vi "LVClass_SlopesPostProcessList GetParameter_DoublePassage.vi"(0 "SlopesPostProcessorList in":refnum<class "SlopesPostProcessorList.lvclass">, 5 "Position":u32, 11 "error in (no error)":errorcluster) -> (4 "SlopesPostProcessorList out":refnum<class "SlopesPostProcessorList.lvclass">, 8 "doublePath":T1, 15 "error out":errorcluster)   [LabVIEW 2020, in "SlopesPostProcessorList.lvclass"]
doc: "Get parameters of the DoublePath processor.\n\n--------------------------------------------------------------------------------\n\n<B>SlopesPostProcessorListIn </B> : SlopesPostProcessorList object.\n<B>SlopesPostProcessorListOut </B> : SlopesPostProcessorList object.\n<B>position </B> : Position of the processor in the SlopesPostProcessorList.\n<B>DoublePathActivateOnTilt </B> : State of Double path activation on tilt.\n<B>DoublePathActivateOnCurvature</B> : State of Double path activation on curvature.\n<B>ErrorIn </B> : Error\n<B>ErrorOut </B> : Error\n\n--------------------------------------------------------------------------------"
uses:
  SlopesPostProcessorList.lvclass
  Controls/SlopesPostProcessorList - Double passage.ctl
  SlopesPostProcessorList.lvclass/SlopesPostProcessorList.ctl
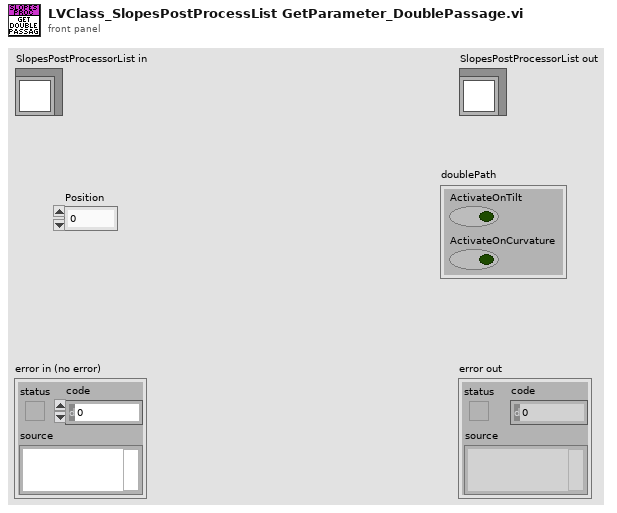
[diagram p1: front panel]
types:
  T1 = typedef "SlopesPostProcessorList - Double passage.ctl" = cluster{"ActivateOnTilt":bool, "ActivateOnCurvature":bool}
  T2 = typedef "ClassID.ctl" = i64
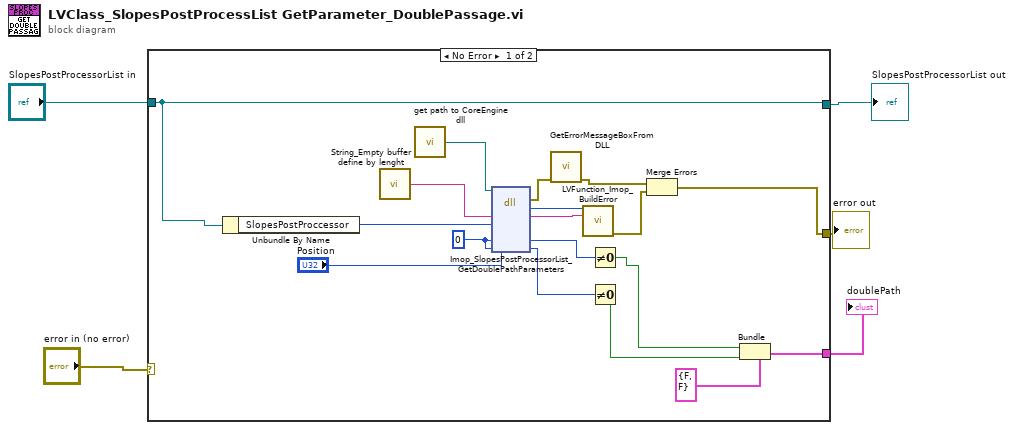
[diagram p0: block diagram]
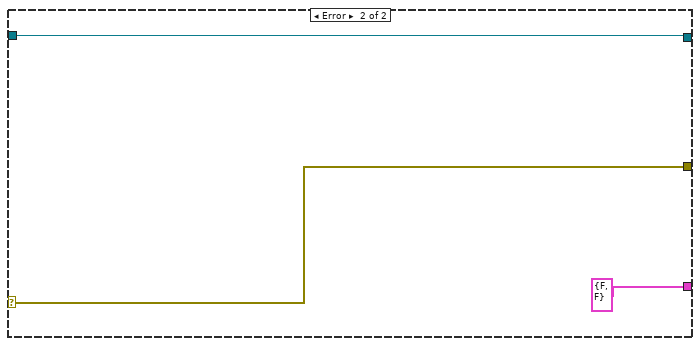
[diagram p2: hidden frame]
diagram:
  n1 = case shown="No Error" "error in (no error)" {
    selector: "error in (no error)" -> [_ w25]
    tunnel: "SlopesPostProcessorList in" -> [w18 w26]
    tunnel: [w18 w26] -> w3
    tunnel: [w10 w25] -> w2
    tunnel: [w7 T1 {"ActivateOnTilt"=FALSE, "ActivateOnCurvature"=FALSE} ("doublePassage")] -> w1
    frame No Error {
      w16 = u8 0 ("doublePassageActivateOnTilt")
      n2 = Unbundle By Name(w18) -> ("SlopesPostProccessor"=w17:T2)
      n3 = call "String_Empty buffer define by lenght.vi"() -> ("Empty buffer"=w23:string)  [unwired: 1 in]
      n4 = call "get path to CoreEngine dll.vi"() -> ("path to wavekit library"=w20:path)  [unwired: 14 in, 1 out]
      n5 = dll-call lib="D:/soft/HASO_v3/SVN_trunk/ImOpCoreEngine4_LV2011/DLLs/c_interface_vc100.dll" fn="Imop_SlopesPostProcessorList_GetDoublePathParameters"(path in=w20, "message"=w23, "objet"=w17, "Position"="Position", "doublePassageActivateOnTilt"=w16, "doublePassageActivateOnCurvature"=w16) -> (error out=w19:errorcluster, "return type"=w21:i32, "message"=w22:string, "doublePassageActivateOnTilt"=w15:u8, "doublePassageActivateOnCurvature"=w14:u8)  [unwired: 4 in, 1 out]
      n6 = call "GetErrorMessageBoxFromDLL.vi"("error IN"=w19) -> ("error OUT"=w12:errorcluster)  [unwired: 10 in]
      n7 = call "LVFunction_Imop_BuildError.vi"("code"=w21, "String to Prepend to source (\"\")"=w22) -> ("error out"=w11:errorcluster)  [unwired: 13 in]
      n8 = Not Equal To 0?(x=w15) -> (x != 0?=w9:bool)
      n9 = Not Equal To 0?(x=w14) -> (x != 0?=w8:bool)
      n10 = Merge Errors(w12, w11) -> (w10:errorcluster)
      n11 = Bundle(cluster=T1 {"ActivateOnTilt"=FALSE, "ActivateOnCurvature"=FALSE} ("doublePassage"), "ActivateOnTilt"=w9, "ActivateOnCurvature"=w8) -> (w7:T1)
    }
    frame Error {
    }
  }
  "error out" <- w2
  "SlopesPostProcessorList out" <- w3
  "doublePath" <- w1
